vi "Handle TCP Connection.vi"(4 "Remote Port":u16, 6 "Remote Host":string, 7 "TCPMessageAPI":refnum<class "TCPMessageAPI.lvclass">, 8 "error in (no error)":errorcluster, 9 "Node ID":u32, 10 "Connection State":T1, 11 "VectoTCPConnectionHandler in":refnum<class "VectoTCPConnectionHandler.lvclass">) -> (0 "error out":errorcluster, 3 "VectoTCPConnectionHandler out":refnum<class "VectoTCPConnectionHandler.lvclass">)   [LabVIEW 2020, in "Vecto.lvlib" / "VectoTCPConnectionHandler.lvclass"]
uses:
  VectoTCPConnectionHandler.lvclass
  VectoService/VectoInfo.lvclass
  Connection Type.ctl
  Vecto.lvlib
  Connection Info.ctl
  Connection State.ctl
  TCPMessaging/TCPMessaging.lvclass
  TCPMessageService/TCPMessageAPI.lvclass
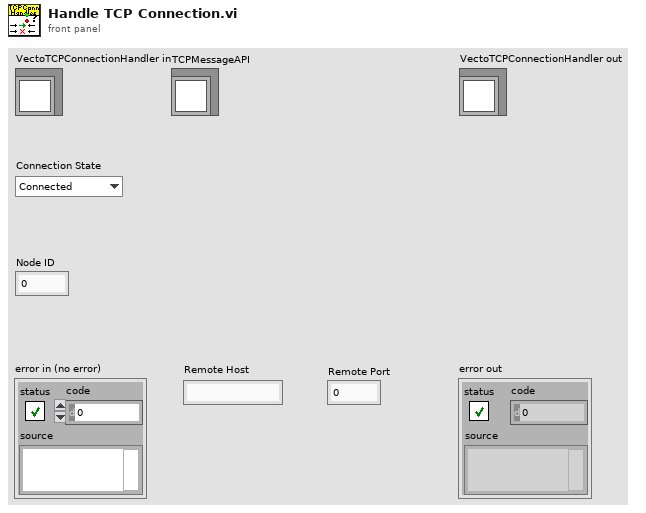
[diagram p1: front panel]
types:
  T1 = typedef "Vecto.lvlib/Connection State.ctl" = enum16{"Connected", "Disconnected"}
  T2 = typedef "Vecto.lvlib/Connection Info.ctl" = cluster{"Name":string, "Type":T3, "RXCount":i32, "TXCount":i32, "Connected":bool, "RemoteIP":u32, "RemotePort":u16, "LocalPort":u16, "Node ID":u32}
  T3 = typedef "Vecto.lvlib/Connection Type.ctl" = enum16{"TCP", "Telemetry", "Discovery", "HTTP"}
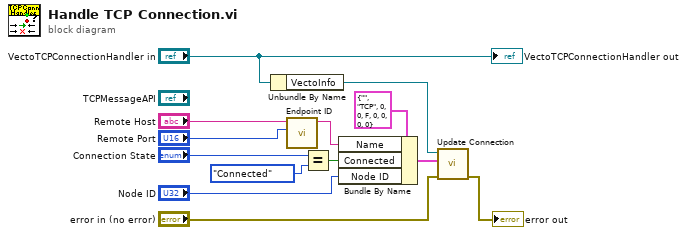
[diagram p0: block diagram]
diagram:
  n1 = Unbundle By Name("VectoTCPConnectionHandler in") -> ("VectoInfo"=w12:refnum<class "VectoInfo.lvclass">)
  n2 = call "Endpoint ID.vi"("Remote Port"="Remote Port", "Remote Address"="Remote Host") -> ("Endpoint ID"=w3:string)  [unwired: 9 in]
  n3 = Equal?(x="Connection State", y=Connection_State."Connected") -> (x = y?=w7:bool)
  n4 = Bundle By Name(cluster=T2 {"Name"="", "Type"=enum."TCP", "RXCount"=0, "TXCount"=0, "Connected"=FALSE, "RemoteIP"=0, "RemotePort"=0, "LocalPort"=0, "Node ID"=0} ("Connection Info"), "Name"=w3, "Connected"=w7, "Node ID"="Node ID") -> (w10:T2)
  n5 = call "Update Connection.vi"("error in (no error)"="error in (no error)", "Connection Info"=w10, "VectoService in"=w12) -> ("error out"=→"error out":errorcluster)  [unwired: 7 in, 1 out]
  "VectoTCPConnectionHandler out" <- "VectoTCPConnectionHandler in"
